vi "Network Engine.vi"() -> ()   [LabVIEW 2013, in "Control Addon Engine.lvlib"]
uses:
  Control Addon Engine.lvlib
  Types/RT Configuration.ctl
  Shared/Types/Gain Schedule.ctl
  Shared/Types/Compiled Settings.ctl
  Shared/Types/Compiled PID Settings.ctl
  <vilib>/NI Veristand/Custom Device API/Block Data Reference.ctl
  <vilib>/NI Veristand/Custom Device API/Data Reference.ctl
  Shared/Types/Compiled Industrial Settings.ctl
  Shared/Types/Compiled Industrial Parameters.ctl
  Stop FG/Stop Global Commands.ctl
  STM API/STM Comm Close All Connections.vi
  STM API/STM Comm Lookup Table_Actions.vi
  Inline Async API/Triggering/Wait on Start Trigger.vi
  STM API/STM Comm Lookup Table_Initialize.vi
  Stop FG/Initialize Global Stop.vi
  Error Handling API/SubVIs/Report Error to Process.vi
  <userlib>/STM/STM Read Meta Data.vi
  <userlib>/STM/TCP/STM Read Meta Data (TCP Ref).vi
  <vilib>/NI Veristand/Custom Device Tools/Custom Device Utility Library/NI VeriStand - Print Debug String.vi
  Stop FG/Stop FG.lvlib
  STM API/STM.lvlib
  Shared/Control Addon Shared.lvlib
  <vilib>/NI VeriStand/Custom Device API/Custom Device API.lvlib
panel:
  out "error out":errorcluster
  in  "stop":bool
  in  "error in (no error)":errorcluster
  in  "Parameters":T1 {"Config"."Industrial Settings"."Write Refs"."Data Reference" format="%.0x"; "Config"."Industrial Settings"."Read Refs"."Data Reference" format="%.0x"; "Config"."PID Settings"."Read Refs"."Data Reference" format="%.0x"; "Config"."PID Settings"."Write Refs"."Data Reference" format="%.0x"}
  in  "Parent":string
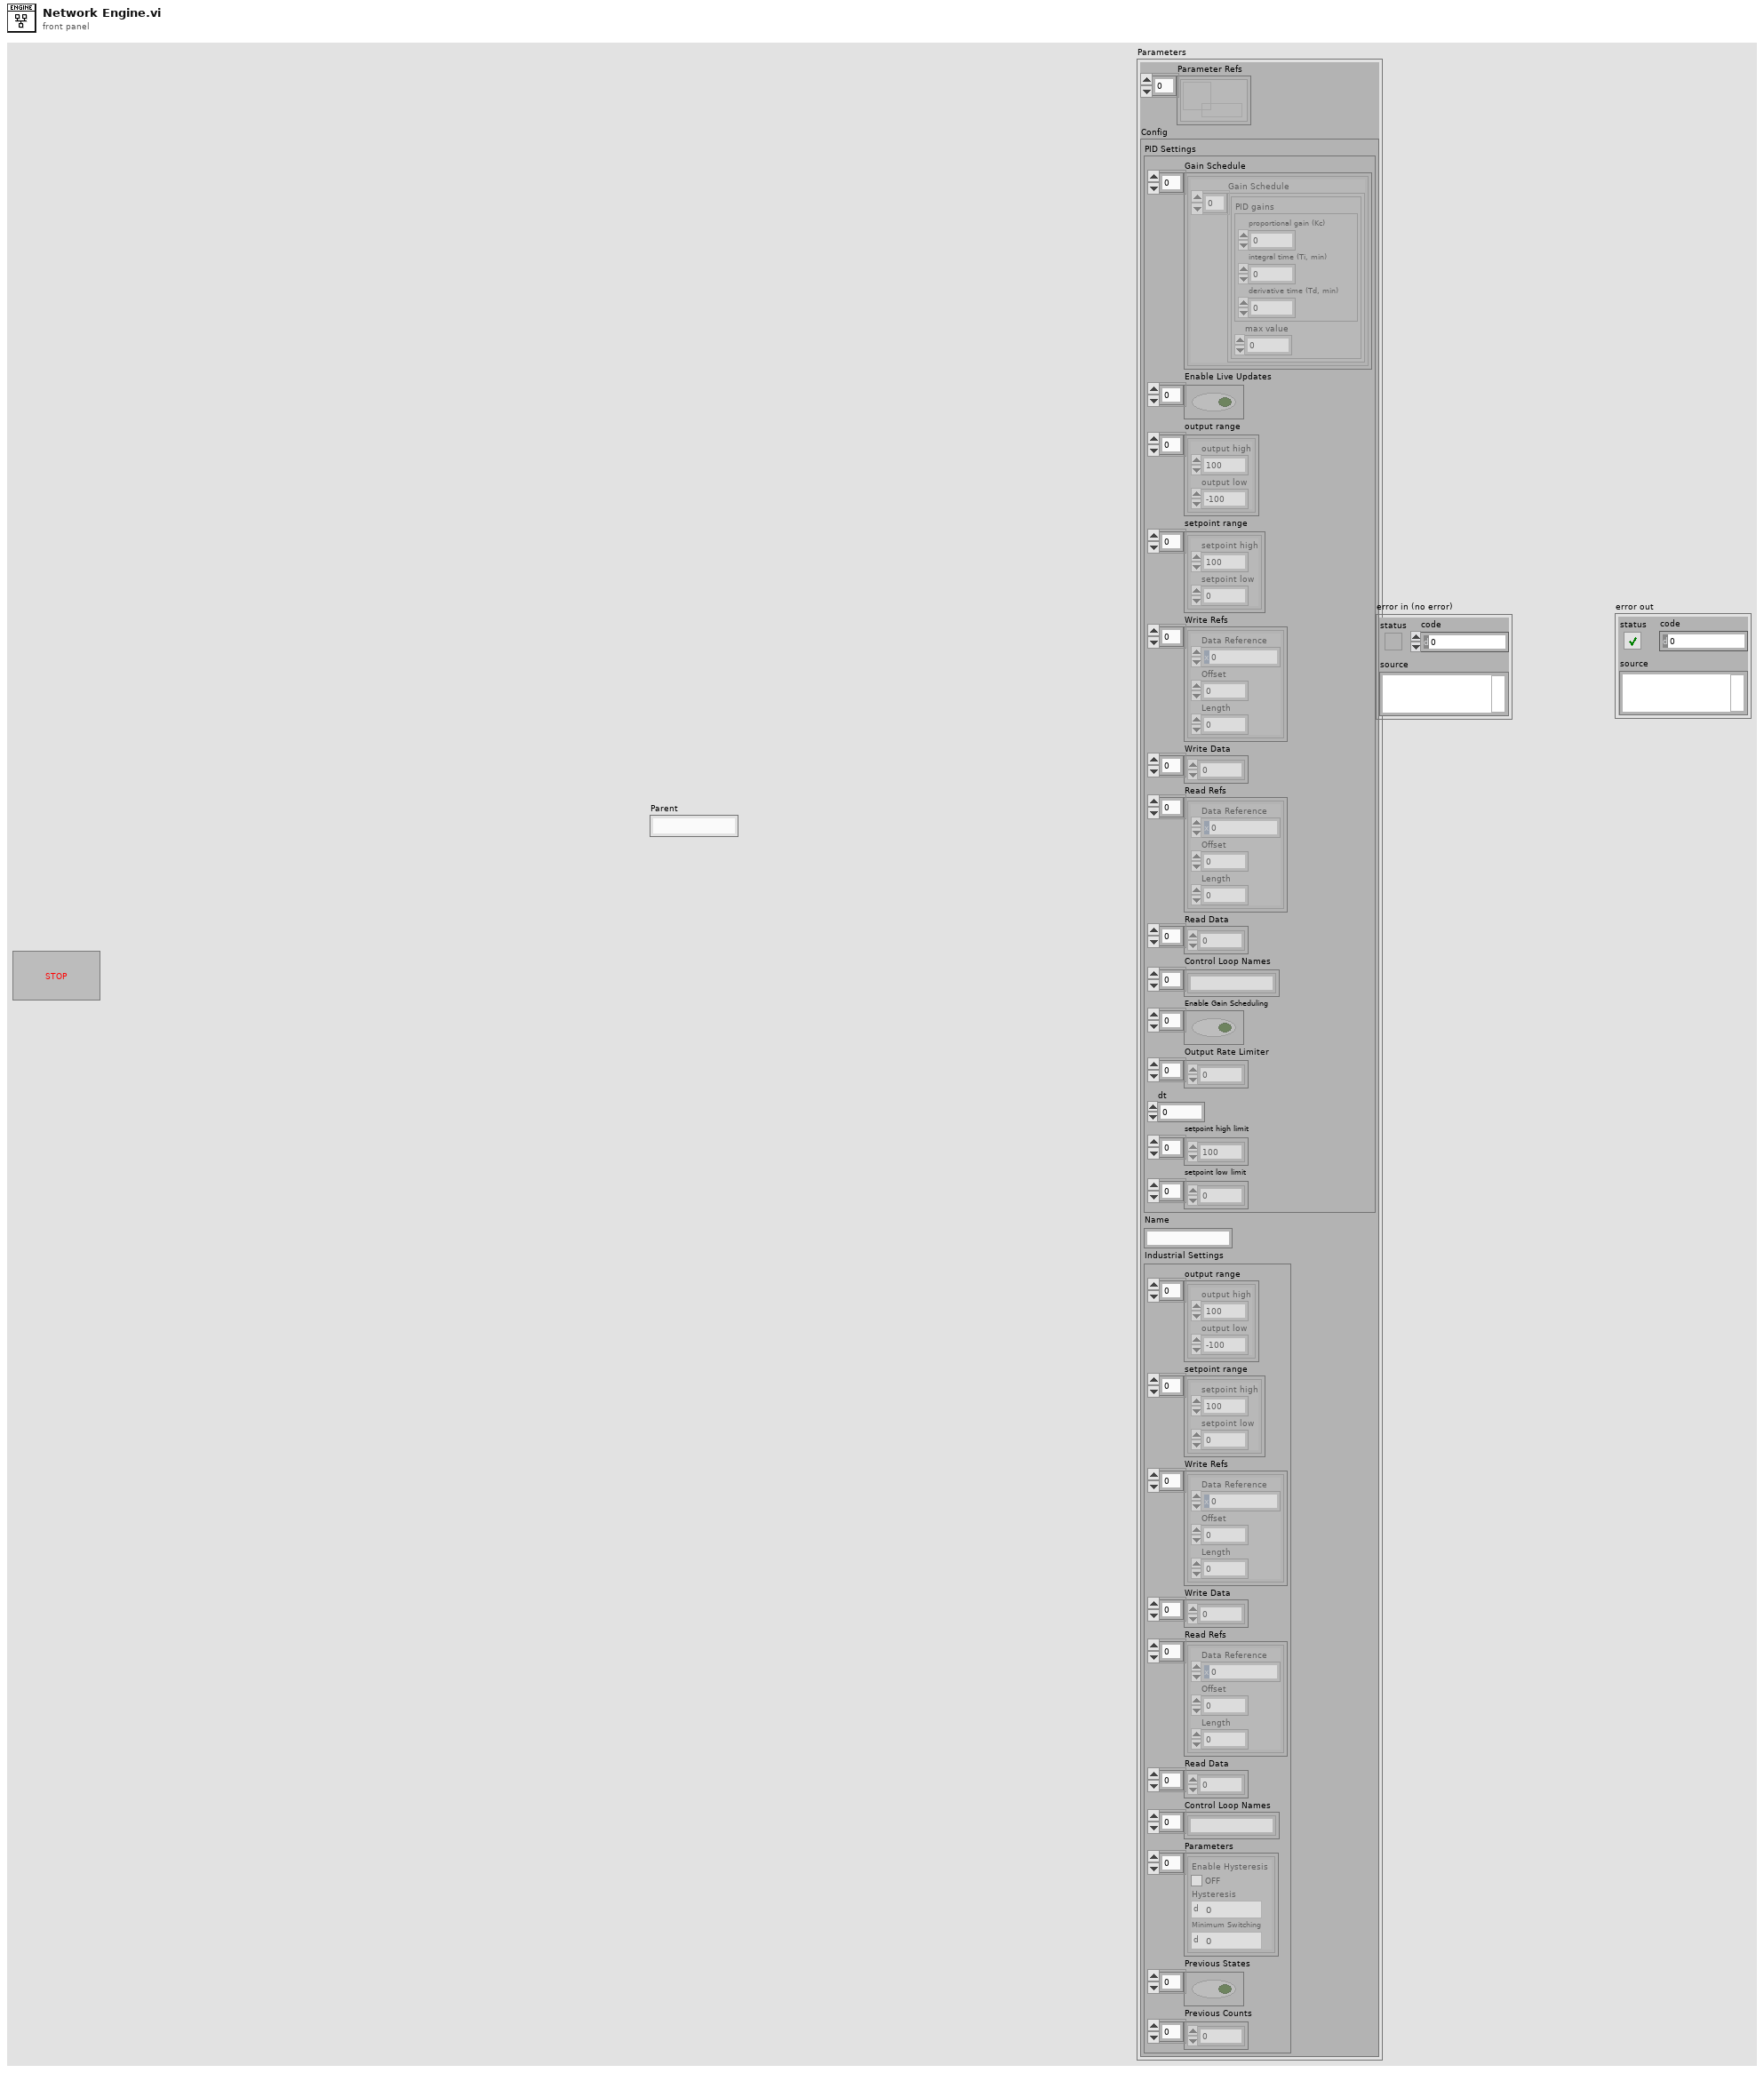
[diagram p1: front panel]
types:
  T1 = typedef "Control Addon Engine.lvlib/RT Configuration.ctl" = cluster{"Parameter Refs":refnum<data-value>[], "Config":T2}
  T2 = typedef "Control Addon Shared.lvlib/Compiled Settings.ctl" = cluster{"PID Settings":T3, "Name":string, "Industrial Settings":T7}
  T3 = typedef "Control Addon Shared.lvlib/Compiled PID Settings.ctl" = cluster{"Gain Schedule":T4[], "Enable Live Updates":bool[], "output range":cluster{"output high":dbl, "output low":dbl}[], "setpoint range":cluster{"setpoint high":dbl, "setpoint low":dbl}[], "Write Refs":T5[], "Write Data":dbl[], "Read Refs":T5[], "Read Data":dbl[], "Control Loop Names":string[], "Enable Gain Scheduling":bool[], "Output Rate Limiter":dbl[], "dt":dbl, "setpoint high limit":dbl[], "setpoint low limit":dbl[]}
  T4 = typedef "Control Addon Shared.lvlib/Gain Schedule.ctl" = cluster{"Gain Schedule":cluster{"PID gains":cluster{"proportional gain (Kc)":dbl, "integral time (Ti, min)":dbl, "derivative time (Td, min)":dbl}, "max value":dbl}[]}
  T5 = typedef "Custom Device API.lvlib/Block Data Reference.ctl" = cluster{"Data Reference":T6, "Offset":i32, "Length":i32}
  T6 = typedef "Custom Device API.lvlib/Data Reference.ctl" = i32
  T7 = typedef "Control Addon Shared.lvlib/Compiled Industrial Settings.ctl" = cluster{"output range":cluster{"output high":dbl, "output low":dbl}[], "setpoint range":cluster{"setpoint high":dbl, "setpoint low":dbl}[], "Write Refs":T5[], "Write Data":dbl[], "Read Refs":T5[], "Read Data":dbl[], "Control Loop Names":string[], "Parameters":T8[], "Previous States":bool[], "Previous Counts":u64[]}
  T8 = typedef "Control Addon Shared.lvlib/Compiled Industrial Parameters.ctl" = cluster{"Enable Hysteresis":bool, "Hysteresis":dbl, "Minimum Switching":u64}
  T9 = typedef "Control Addon Engine.lvlib/Inline Async API.lvlib/Engine State Variables.ctl" = cluster{"Stop":T10, "Top VI":refnum<vi>, "Name":string, "listener ID":refnum<k5>, "TCP Ref":T11}
  T10 = typedef "Control Addon Engine.lvlib/Stop FG.lvlib/Stop Global Ref.ctl" = refnum<vi>
  T11 = typedef "Control Addon Engine.lvlib/STM.lvlib/STM Comm Lookup Table_Ref.ctl" = refnum<vi>
  T12 = typedef "Control Addon Engine.lvlib/Stop FG.lvlib/Stop Global Commands.ctl" = enum16{"Write", "Read", "Reset"}
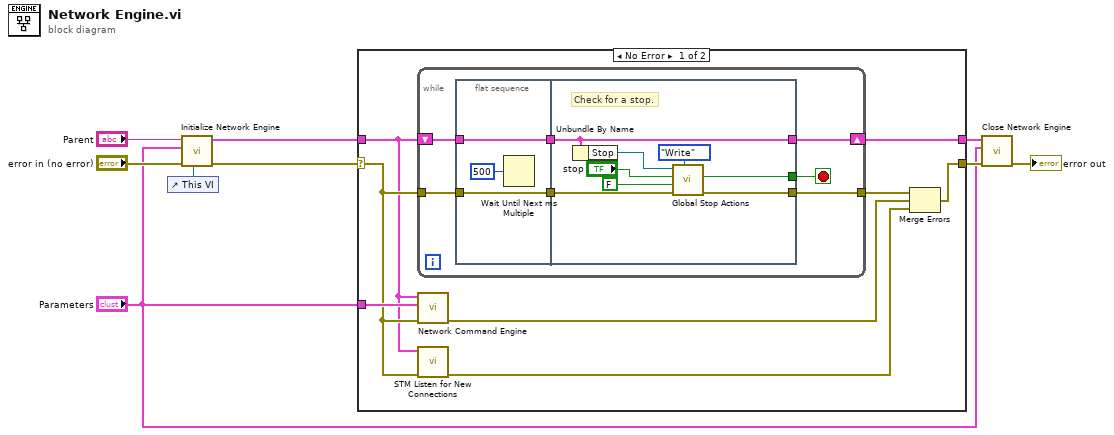
[diagram p0: block diagram]
diagram:
  n1 = control-ref of="This VI"() -> (w4:refnum<vi>)
  n2 = call "Initialize Network Engine.vi"("VI in"=w4, "error in (no error)"="error in (no error)", "Parameters"="Parameters", "Parent"="Parent") -> ("error out"=w2:errorcluster, "State Variables"=w8:T9)  [unwired: 6 in]
  n3 = case shown="No Error" w2 {
    selector: w2 -> [w12 w37]
    tunnel: w8 -> [w11 w36]
    tunnel: [w17 w36] -> w7
    tunnel: "Parameters" -> [w15 _]
    tunnel: [w14 w37] -> w3
    frame No Error {
      n4 = while {
        tunnel: w12 -> [w23]
        tunnel: [w18] -> w16
        shift-right: [w19] -> w17
        shift-left: w11 -> [w21]
        stop <- w24 stop-if-true
        n5 = flat-sequence {
          tunnel: w23 -> [w27]
          tunnel: [w27] -> w22
          tunnel: w21 -> [w25]
          tunnel: [w25] -> w20
          tunnel: [w32] -> w24
          tunnel: [w33] -> w18
          tunnel: w22 -> [w34]
          tunnel: w20 -> [w35]
          tunnel: [w35] -> w19
          frame #0 {
            n6 = Wait Until Next ms Multiple(millisecond multiple=u32 500) -> ()  [unwired: 1 out]
          }
          frame #1 {
            # "Check for a stop."
            n7 = Unbundle By Name(w35) -> ("Stop"=w31:T10)
            n8 = call "Global Stop Actions.vi"("Command"=Stop_Global_Commands."Write", "error in (no error)"=w34, "Stop on Error?"=FALSE, "Stop?"="stop", "vi reference"=w31) -> ("error out"=w33:errorcluster, "Latched Stop"=w32:bool)  [unwired: 4 in, 1 out]
          }
        }
      }
      n9 = call "Network Command Engine.vi"("error in (no error)"=w12, "Parameters"=w15, "State Variables"=w11) -> ("error out"=w13:errorcluster)  [unwired: 8 in]
      n10 = call "STM Listen for New Connections.vi"("error in (no error)"=w12, "State Variables"=w11) -> ("error out"=w10:errorcluster)  [unwired: 9 in]
      n11 = Merge Errors(w16, w13, w10) -> (w14:errorcluster)
    }
    frame Error {
    }
  }
  n12 = call "Close Network Engine.vi"("error in (no error)"=w3, "Parameters"="Parameters", "State Variables"=w7) -> ("error out"=→"error out":errorcluster)  [unwired: 8 in]
